vi "Speak text.vi"(1 "Text to speak":string="testing 1 2 3") -> (0 "Error out":errorcluster)   [LabVIEW 2013]
uses:
  System.Speech
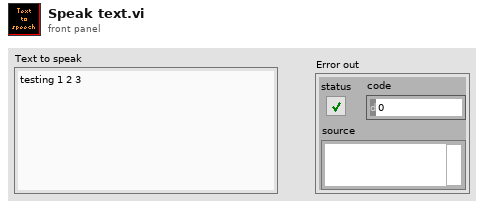
[diagram p1: front panel]
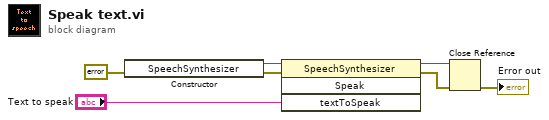
[diagram p0: block diagram]
diagram:
  n1 = constructor class="SpeechSynthesizer"(error in=errorcluster {"status"=FALSE, "code"=0, "source"=""} ("error in (no error)")) -> (reference out=w4:refnum<k24>, error out=w5:errorcluster)  [unwired: 2 in, 1 out]
  n2 = invoke class="SpeechSynthesizer" method="Speak"(reference=w4, error in=w5, "textToSpeak"="Text to speak") -> (reference out=w3:refnum<k24>, error out=w2:errorcluster)  [unwired: 1 in, 2 out]
  n3 = Close Reference(reference=w3, error in (no error)=w2) -> (error out=→"Error out":errorcluster)
